vi "20T_Merge_Cluster.vi"(1 "VTI Control":T2={"Clamp"=FALSE, "Switch Heater"=FALSE, "Go to Zero"=FALSE, "Go to Set"=FALSE, "Go to Hold"=FALSE, "Setpoint (T)"=3.4572, "Rate (T/min)"=0.0, "Set Rate"=FALSE} {"Rate (T/min)" format="%6_5f"; "Setpoint (T)" format="%#4_5f"}, 2 "VTI Status":T3={"Clamped"=FALSE, "Quenched"=FALSE, "Rate limit"=FALSE, "Persistent"=TRUE, "Hold"=TRUE, "Set"=FALSE, "Zero"=FALSE, "Magnet (T)"=0.0, "Leads (T)"=0.0, "Magnet T (K)"=0.0, "Switch"=FALSE} {"Magnet T (K)" format="%#4_5f"; "Leads (T)" format="%6_5f"}) -> (0 "20 T Magnet control":T1={"Clamp"=FALSE, "Switch Heater"=FALSE, "Go to Zero"=FALSE, "Go to set"=FALSE, "Go to Hold"=FALSE, "Clamped"=FALSE, "Quenched"=FALSE, "Rate limit"=FALSE, "Persistent"=FALSE, "Hold"=FALSE, "Set"=FALSE, "Zero"=FALSE, "Magnet (T)"=0.0, "Leads (T)"=0.0, "Magnet T (K)"=3.4572, "Switch"=FALSE, "Target (T)"=3.4572, "Setpoint (T)"=3.4572, "Rate (T/min)"=0.0, "Switch Heater 2"=FALSE, "Set Rate"=FALSE} {"Rate (T/min)" format="%6_5f"; "Setpoint (T)" format="%6_5f"; "Target (T)" format="%#4_5f"; "Magnet T (K)" format="%#4_5f"; "Leads (T)" format="%6_5f"})   [LabVIEW 2018]
uses:
  Gustav/20T_Status.ctl
  Gustav/20T_Control.ctl
  Gustav/20T_Cluster.ctl
panel:
  # "20 T"
  # "20 T"
  # "20 T"
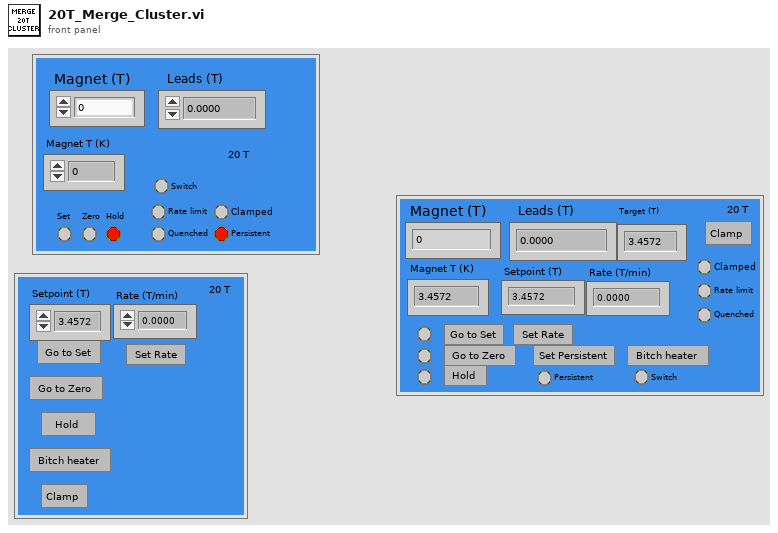
[diagram p1: front panel]
types:
  T1 = typedef "20T_Cluster.ctl" = cluster{"Clamp":bool, "Switch Heater":bool, "Go to Zero":bool, "Go to set":bool, "Go to Hold":bool, "Clamped":bool, "Quenched":bool, "Rate limit":bool, "Persistent":bool, "Hold":bool, "Set":bool, "Zero":bool, "Magnet (T)":dbl, "Leads (T)":dbl, "Magnet T (K)":dbl, "Switch":bool, "Target (T)":dbl, "Setpoint (T)":dbl, "Rate (T/min)":dbl, "Switch Heater 2":bool, "Set Rate":bool}
  T2 = typedef "20T_Control.ctl" = cluster{"Clamp":bool, "Switch Heater":bool, "Go to Zero":bool, "Go to Set":bool, "Go to Hold":bool, "Setpoint (T)":dbl, "Rate (T/min)":dbl, "Set Rate":bool}
  T3 = typedef "20T_Status.ctl" = cluster{"Clamped":bool, "Quenched":bool, "Rate limit":bool, "Persistent":bool, "Hold":bool, "Set":bool, "Zero":bool, "Magnet (T)":dbl, "Leads (T)":dbl, "Magnet T (K)":dbl, "Switch":bool}
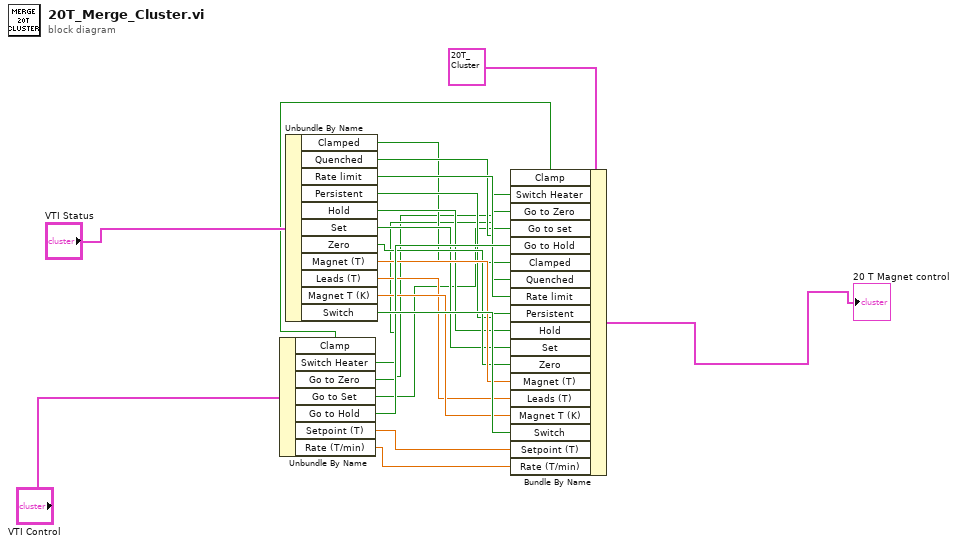
[diagram p0: block diagram]
diagram:
  n1 = Unbundle By Name("VTI Control") -> ("Clamp"=w5:bool, "Switch Heater"=w4:bool, "Go to Zero"=w3:bool, "Go to Set"=w2:bool, "Go to Hold"=w16:bool, "Setpoint (T)"=w18:dbl, "Rate (T/min)"=w1:dbl)
  n2 = Unbundle By Name("VTI Status") -> ("Clamped"=w6:bool, "Quenched"=w7:bool, "Rate limit"=w9:bool, "Persistent"=w8:bool, "Hold"=w10:bool, "Set"=w11:bool, "Zero"=w12:bool, "Magnet (T)"=w13:dbl, "Leads (T)"=w14:dbl, "Magnet T (K)"=w15:dbl, "Switch"=w17:bool)
  n3 = Bundle By Name(cluster=T1 {"Clamp"=FALSE, "Switch Heater"=FALSE, "Go to Zero"=FALSE, "Go to set"=FALSE, "Go to Hold"=FALSE, "Clamped"=TRUE, "Quenched"=TRUE, "Rate limit"=FALSE, "Persistent"=FALSE, "Hold"=FALSE, "Set"=FALSE, "Zero"=FALSE, "Magnet (T)"=0.0, "Leads (T)"=0.0, "Magnet T (K)"=3.4572, "Switch"=FALSE, "Target (T)"=3.4572, "Setpoint (T)"=3.4572, "Rate (T/min)"=0.0, "Switch Heater 2"=FALSE, "Set Rate"=FALSE} ("VTI Cluster 2"), "Clamp"=w5, "Switch Heater"=w4, "Go to Zero"=w3, "Go to set"=w2, "Go to Hold"=w16, "Clamped"=w6, "Quenched"=w7, "Rate limit"=w9, "Persistent"=w8, "Hold"=w10, "Set"=w11, "Zero"=w12, "Magnet (T)"=w13, "Leads (T)"=w14, "Magnet T (K)"=w15, "Switch"=w17, "Setpoint (T)"=w18, "Rate (T/min)"=w1) -> (→"20 T Magnet control":T1)
